vi "CameraSetProperties.vi"(8 "error in (no error)":errorcluster, 10 "set?":bool, 11 "CameraBase in":refnum<class "CameraBase.lvclass">) -> (0 "error out":errorcluster, 2 "cam_params":cluster{"String":string, "value":variant}[](array[cluster]) caption="parameters", 3 "CameraBase out":refnum<class "CameraBase.lvclass">)   [LabVIEW 2010, in "CameraBase.lvclass"]
uses:
  CameraBase.lvclass
panel:
  in  "cancel":bool
  in  "ok":bool
  # "Camera Configuration"
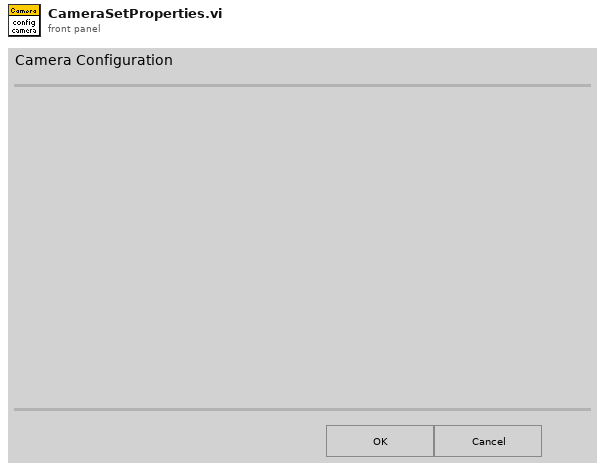
[diagram p1: front panel]
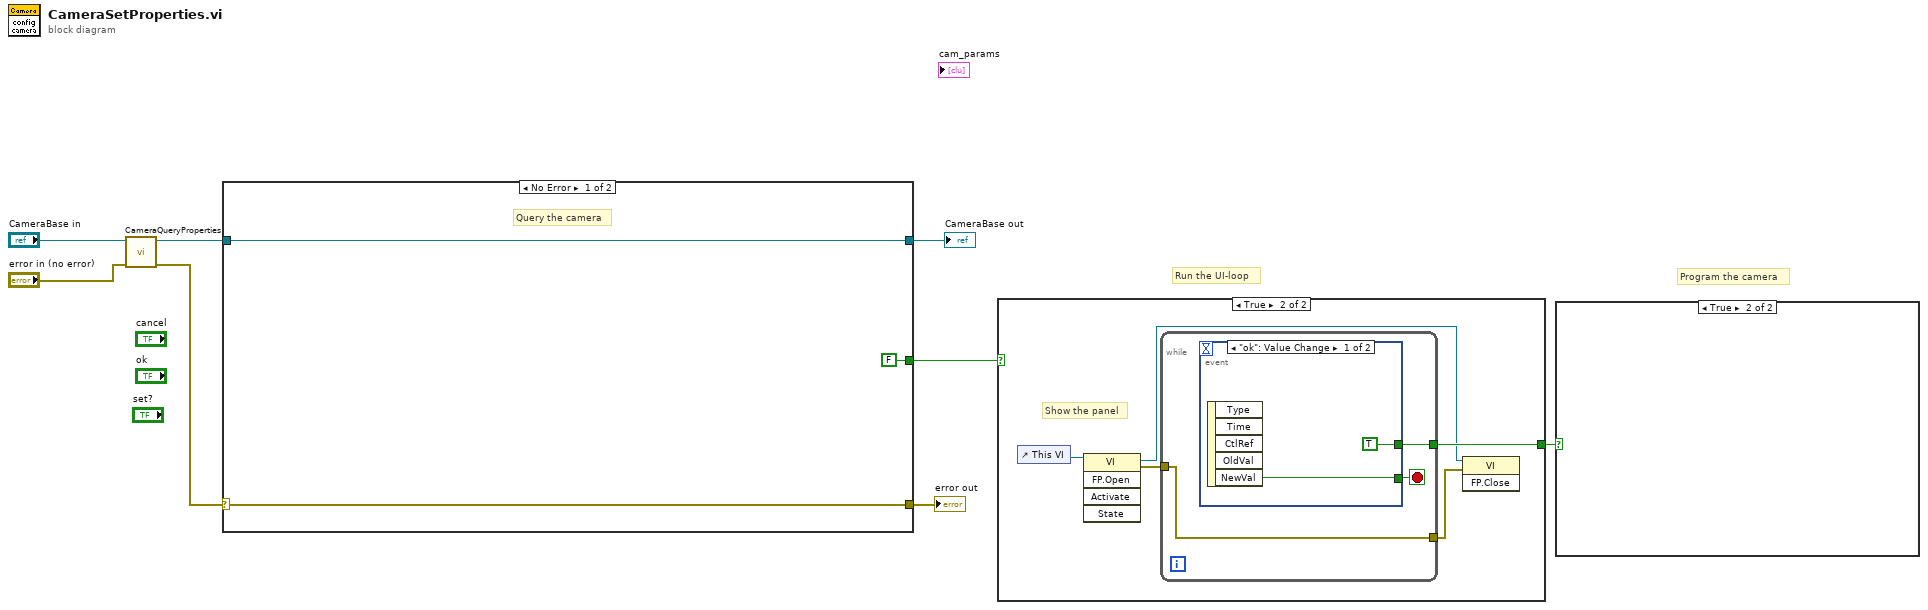
[diagram p0: block diagram]
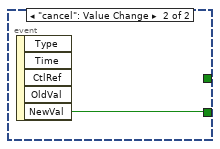
[diagram p4: hidden frame]
diagram:
  # "Program the camera"
  # "Run the UI-loop"
  n1 = call-dynamic "CameraQueryProperties.vi"("error in (no error)"="error in (no error)", "CameraBase in"="CameraBase in") -> ("error out"=w1:errorcluster, "CameraBase out"=w3:refnum<class "CameraBase.lvclass">)  [unwired: 5 in, 3 out]
  n2 = case shown="No Error" w1 {
    selector: w1 -> [w11 w13]
    tunnel: [w11 w13] -> w8
    tunnel: [w10 w12] -> w6
    tunnel: w3 -> [w10 w12]
    tunnel: [FALSE ("set?") _] -> w7
    frame No Error {
      # "Query the camera"
    }
    frame Error {
    }
  }
  "error out" <- w8
  "CameraBase out" <- w6
  n3 = case shown="True" w7 {
    tunnel: [_ w16] -> w5
    frame False {
    }
    frame True {
      # "Show the panel"
      n4 = control-ref of="This VI"() -> (w18:refnum<vi>)
      n5 = invoke class="VI" method="FP.Open"(reference=w18) -> (reference out=w14:refnum<vi>, error out=w17:errorcluster)  [unwired: 4 in, 3 out]
      n6 = while {
        tunnel: w17 -> [w19]
        tunnel: [w20] -> w16
        tunnel: [w19] -> w15
        stop <- w21 stop-if-true
        n7 = event shown="[0] \"ok\": Value Change" {
          selector: _ -> [_ _]
          dyn-events: _ -> [_ _]
          timeout: _ -> [_ _]
          tunnel: [w23 w24] -> w21
          tunnel: [TRUE ("ok") _] -> w20
          event "ok": Value Change {
            n8 = event-data() -> ("NewVal"=w23:bool)  [unwired: 1 in, 4 out]
          }
          event "cancel": Value Change {
            n9 = event-data() -> ("NewVal"=w24:bool)  [unwired: 1 in, 4 out]
          }
        }
      }
      n10 = invoke class="VI" method="FP.Close"(reference=w14, error in=w15) -> ()  [unwired: 1 in, 3 out]
    }
  }
  n11 = case shown="True" w5 {
    frame False {
    }
    frame True {
    }
  }
